vi "GetShotDistance(SubVI).vi"(10 "Array in":i32[](array[numeric]), 11 "Gun Fire Button":bool) -> (0 "Current Dist":i16, 3 "Numeric":i16)   [LabVIEW 2017]
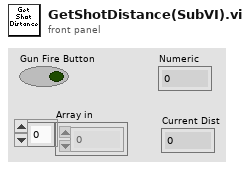
[diagram p1: front panel]
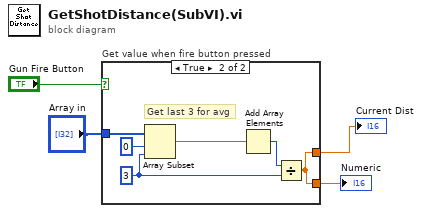
[diagram p0: block diagram]
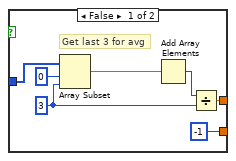
[diagram p2: hidden frame]
diagram:
  n1 = case "Get value when fire button pressed" shown="True" "Gun Fire Button" {
    tunnel: "Array in" -> [w6 w16]
    tunnel: [-1 w12] -> w3
    tunnel: [w5 w12] -> w1
    frame False {
      w7 = 3
      # "Get last 3 for avg"
      n2 = Array Subset(array=w6, index=0, length=w7) -> (w9:i32[])
      n3 = Add Array Elements(numeric array=w9) -> (sum=w10:i32)
      n4 = Divide(x=w10, y=w7) -> (x/y=w5:dbl)
    }
    frame True {
      w14 = 3
      # "Get last 3 for avg"
      n5 = Array Subset(array=w16, index=0, length=w14) -> (w15:i32[])
      n6 = Add Array Elements(numeric array=w15) -> (sum=w13:i32)
      n7 = Divide(x=w13, y=w14) -> (x/y=w12:dbl)
    }
  }
  "Numeric" <- w3
  "Current Dist" <- w1
